vi "BusB_Configure Hardware.vi"(8 "error in (no error)":errorcluster, 11 "BusB Visa Resource in":refnum<visa-resource-name>) -> (0 "error out":errorcluster, 3 "BusB Visa Resource out":refnum<visa-resource-name>)   [LabVIEW 2016, in "Impedance Data Acquisition and Decoding.lvlib"]
uses:
  Impedance Data Acquisition and Decoding.lvlib
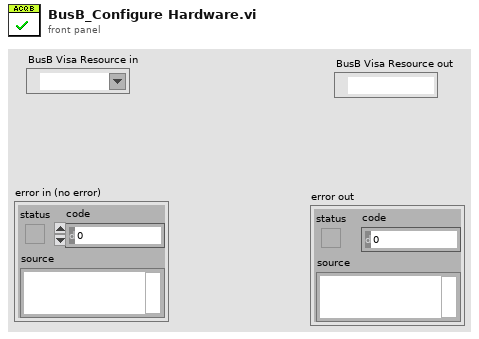
[diagram p1: front panel]
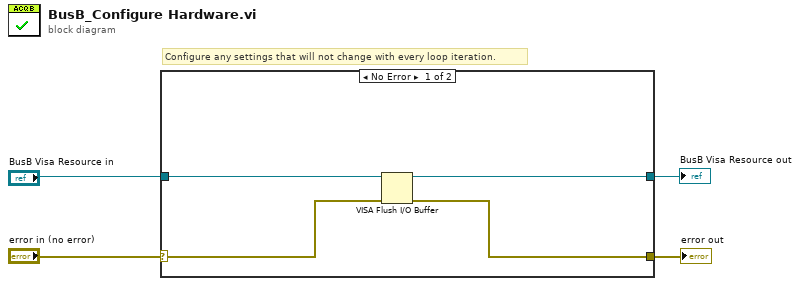
[diagram p0: block diagram]
diagram:
  # "Configure any settings that will not change with every loop iteration."
  n1 = case shown="No Error" "error in (no error)" {
    selector: "error in (no error)" -> [w8 w10]
    tunnel: [w7 w10] -> w3
    tunnel: [w6 w9] -> w2
    tunnel: "BusB Visa Resource in" -> [w5 w9]
    frame No Error {
      n2 = VISA Flush I/O Buffer(VISA resource name=w5, error in (no error)=w8) -> (VISA resource name out=w6:refnum<visa-resource-name>, error out=w7:errorcluster)  [unwired: 1 in]
    }
    frame Error {
    }
  }
  "error out" <- w3
  "BusB Visa Resource out" <- w2
